vi "MCL Init Handle Or Get Existing.vi"() -> (3 "function return":i32)   [LabVIEW 2017, in "Madlib.lvlib"]
doc: "MADLIB_API int MCL_InitHandleOrGetExisting();"
uses:
  Madlib.lvlib
  Madlib.dll
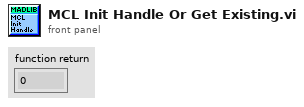
[diagram p1: front panel]
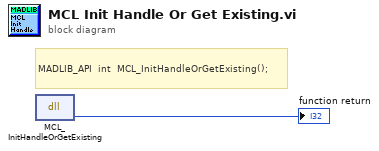
[diagram p0: block diagram]
diagram:
  # "MADLIB_API  int\t\tMCL_InitHandleOrGetExisting();"
  n1 = dll-call lib="C:/Users/francesco/dev/pump-probe/Piezo/lvlib/Madlib.*" fn="MCL_InitHandleOrGetExisting"() -> (→"function return":i32)  [unwired: 3 in, 2 out]
